vi "Prompt for Step--Init UI.vi"(8 "error in (no error)":errorcluster, 10 "Control Ref Map":map{string, refnum<vi>}(c390), 11 "Boolean Assertion in":refnum<class "Boolean Assertion.lvclass">) -> (0 "error out":errorcluster, 3 "Boolean Assertion out":refnum<class "Boolean Assertion.lvclass">)   [LabVIEW 2020, in "MacroAssert.lvlib" / "Boolean Assertion.lvclass"]
doc: "Initializes the user interface within the \"Prompt for Step\" VI."
uses:
  Boolean Assertion.lvclass
  Support/Get Control Reference by Label (1D STR).vi
  <vilib>/Utility/error.llb/Error Cluster From Error Code.vi
  Assertion Step/Assertion Step.lvclass
  MacroAssert.lvlib
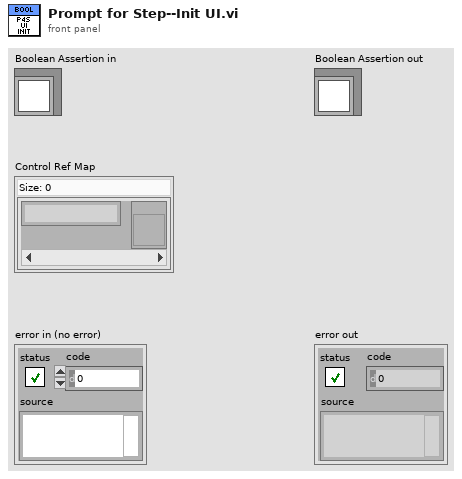
[diagram p1: front panel]
types:
  T1 = typedef "MacroAssert.lvlib/Boolean Assertion.lvclass/Boolean Assertion Type.ctl" = enum16{"Boolean Ctl Value", "Ctl Visible Property", "Ctl is Enabled", "Ctl is Grayed Out", "Ctl Key Focus Property", "Window is in Running Windows", "VI Front Panel is Open"}
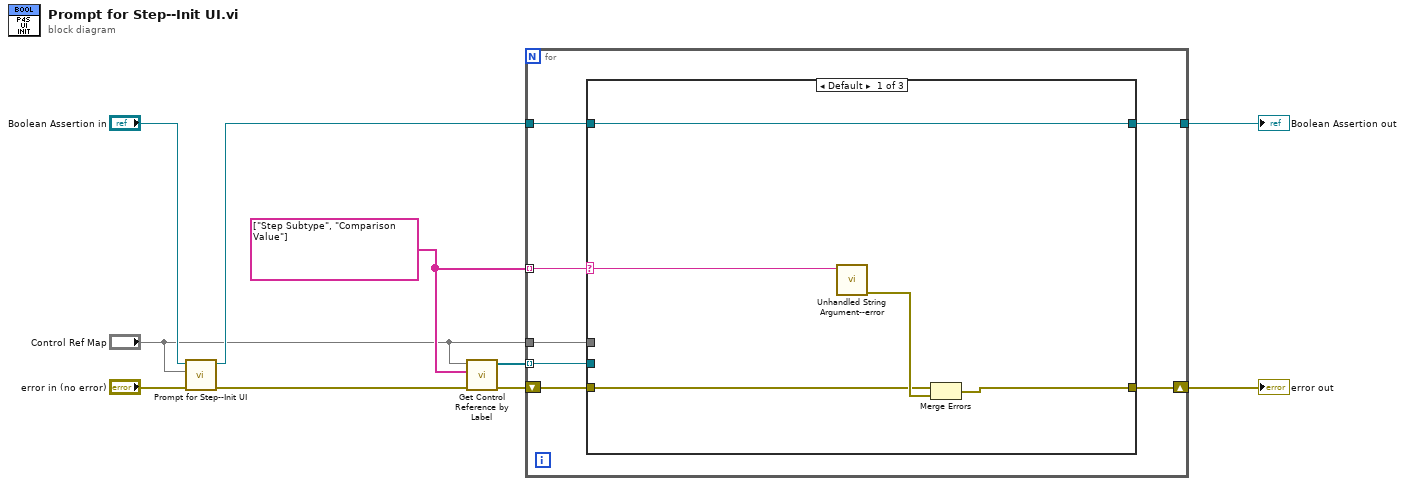
[diagram p0: block diagram]
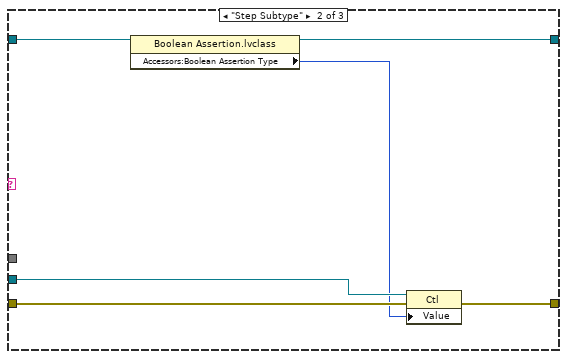
[diagram p2: hidden frame]
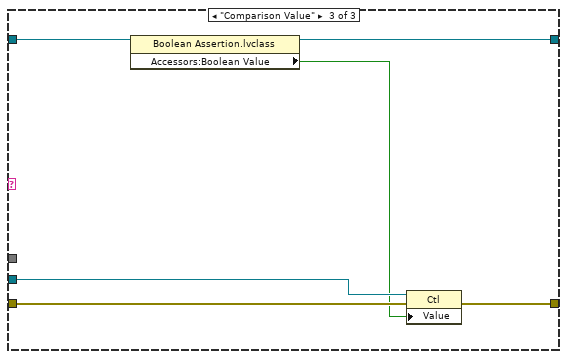
[diagram p3: hidden frame]
diagram:
  w9 = string[] ["Step Subtype", "Comparison Value"]
  n1 = call-parent "Prompt for Step--Init UI.vi"("error in (no error)"="error in (no error)", "Control Ref Map"="Control Ref Map", "Assertion Step in"="Boolean Assertion in") -> ("error out"=w4:errorcluster, "Assertion Step out"=w2:refnum<class "Boolean Assertion.lvclass">)  [unwired: 7 in]
  n2 = call-poly "Get Control Reference by Label.vi"("error in (no error)"=w4, "Control Names"=w9, "Control Ref Map"="Control Ref Map") -> ("error out"=w10:errorcluster, "Control Refs"=w8:refnum<vi>[])  [unwired: 6 in, 1 out]
  n3 = for {
    tunnel: w2 -> [w15]
    tunnel: [w13] -> w6
    tunnel: w9 -> [w16] mode=indexing
    tunnel: w8 -> [w14] mode=indexing
    shift-right: [w12] -> w7
    shift-left: w10 -> [w17]
    tunnel: "Control Ref Map" -> [w11]
    n4 = case shown="Default" w16 {
      selector: w16 -> [w19 _ _]
      tunnel: w17 -> [w21 w25 w31]
      tunnel: w15 -> [w18 w28 w34]
      tunnel: w14 -> [_ w26 w32]
      tunnel: [w18 w27 w33] -> w13
      tunnel: [w20 w23 w29] -> w12
      tunnel: w11 -> [_ _ _]
      frame Default {
        n5 = call "Unhandled String Argument--error.vi"("Argument"=w19) -> ("error out"=w22:errorcluster)  [unwired: 10 in]
        n6 = Merge Errors(w21, w22) -> (w20:errorcluster)
      }
      frame "Step Subtype" {
        n7 = property class="Boolean Assertion.lvclass"(reference=w28) -> (reference out=w27:refnum<class "Boolean Assertion.lvclass">, "Accessors:Boolean Assertion Type"=w24:T1)  [unwired: 1 in, 1 out]
        n8 = property class="Ctl"(reference=w26, error in=w25, "Value"=w24) -> (error out=w23:errorcluster)  [unwired: 1 out]
      }
      frame "Comparison Value" {
        n9 = property class="Boolean Assertion.lvclass"(reference=w34) -> (reference out=w33:refnum<class "Boolean Assertion.lvclass">, "Accessors:Boolean Value"=w30:bool)  [unwired: 1 in, 1 out]
        n10 = property class="Ctl"(reference=w32, error in=w31, "Value"=w30) -> (error out=w29:errorcluster)  [unwired: 1 out]
      }
    }
  }
  "error out" <- w7
  "Boolean Assertion out" <- w6
